vi "Buzzer Pressed.vi"(8 "error in (no error)":errorcluster, 10 "Buzzer":i32, 11 "Controller in":refnum<class "Controller.lvclass">) -> (0 "error out":errorcluster, 3 "Controller out":refnum<class "Controller.lvclass">)   [LabVIEW 2024, in "Controller.lvlib" / "Controller.lvclass"]
uses:
  Controller.lvclass
  Controller.lvclass/Controller.ctl
  MC Prompt/MC Prompt Messages/Contestant Buzzed Msg/Contestant Buzzed Msg.lvclass/Contestant Buzzed Msg.ctl
  <vilib>/ActorFramework/Message Enqueuer/Message Enqueuer.lvclass/Message Enqueuer.ctl
  <vilib>/ActorFramework/Message Enqueuer/Enqueue.vi
  MC Prompt/MC Prompt Messages/Contestant Buzzed Msg/Contestant Buzzed Msg.lvclass
  Contestant/Contestant Messages/Light to Green Msg/Light to Green Msg.lvclass
  <vilib>/ActorFramework/Message Priority Queue/Priority Enqueue.vi
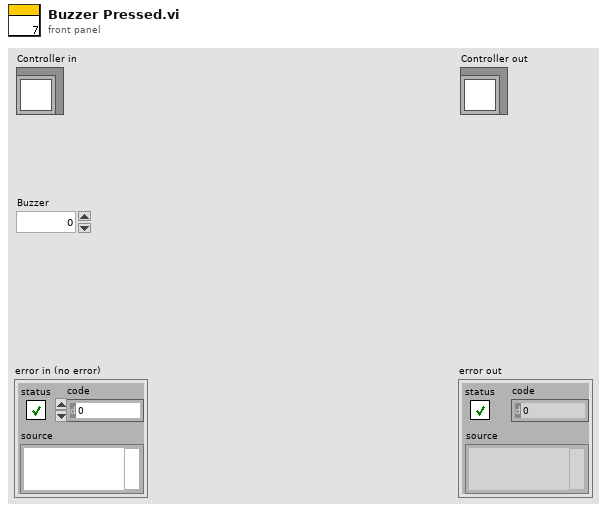
[diagram p1: front panel]
types:
  T1 = map{i32, refnum<class "Message Enqueuer.lvclass">}
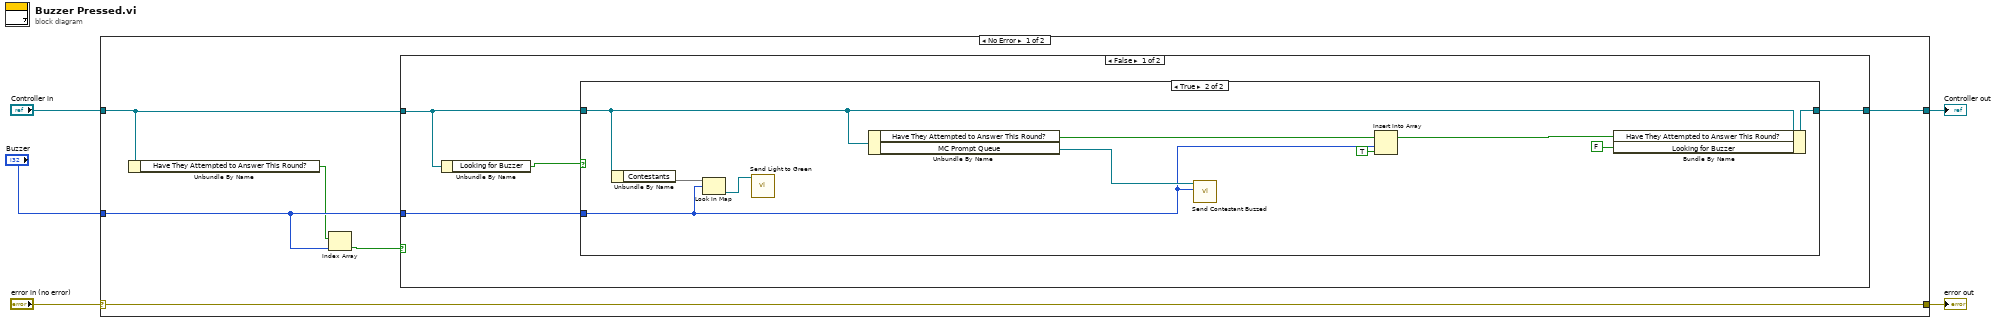
[diagram p0: block diagram]
diagram:
  n1 = case shown="No Error" "error in (no error)" {
    selector: "error in (no error)" -> [w11 w29]
    tunnel: [w11 w29] -> w4
    tunnel: [w10 w28] -> w2
    tunnel: "Controller in" -> [w9 w28]
    tunnel: "Buzzer" -> [w8 _]
    frame No Error {
      n2 = Unbundle By Name(w9) -> ("Have They Attempted to Answer This Round?"=w7:bool[])
      n3 = Index Array(array=w7, index=w8) -> (element=w6:bool)
      n4 = case shown="False" w6 {
        tunnel: [w14 w27] -> w10
        tunnel: w9 -> [w13 w27]
        tunnel: w8 -> [w12 _]
        frame False {
          n5 = Unbundle By Name(w13) -> ("Looking for Buzzer"=w15:bool)
          n6 = case shown="True" w15 {
            tunnel: w12 -> [_ w20]
            tunnel: w13 -> [w16 w23]
            tunnel: [w16 w22] -> w14
            frame False {
            }
            frame True {
              n7 = Unbundle By Name(w23) -> ("Contestants"=w26:T1)
              n8 = Look In Map(map=w26, key=w20) -> (value=w25:refnum<class "Message Enqueuer.lvclass">)  [unwired: 1 in, 1 out]
              n9 = call "Send Light to Green.vi"("Message Enqueuer"=w25) -> ()  [unwired: 9 in, 2 out]
              n10 = Unbundle By Name(w23) -> ("Have They Attempted to Answer This Round?"=w21:bool[], "MC Prompt Queue"=w24:refnum<class "Message Enqueuer.lvclass">)
              n11 = call "Send Contestant Buzzed.vi"("Contestant"=w20, "Message Enqueuer"=w24) -> ()  [unwired: 8 in, 2 out]
              n12 = Insert Into Array(array=w21, index=w20, new element=TRUE ("new element/subarray")) -> (w18:bool[])
              n13 = Bundle By Name(cluster=w23, "Have They Attempted to Answer This Round?"=w18, "Looking for Buzzer"=FALSE) -> (w22:refnum<class "Controller.lvclass">)
            }
          }
        }
        frame True {
        }
      }
    }
    frame Error {
    }
  }
  "error out" <- w4
  "Controller out" <- w2
